vi "Add Lockin Comments.vi"(7 "error in (no error)":errorcluster, 10 "Control Experiment":refnum<class "Control Experiment.lvclass">) -> (0 "error out":errorcluster, 3 "Control Experiment out":refnum<class "Control Experiment.lvclass">)   [LabVIEW 2016, in "Control Experiment.lvclass"]
uses:
  Control Experiment.lvclass
  Typedefs/Lockin Configuration--cluster.ctl
  <userlib>/LevyLab/Lockin-Multichannel/Instrument.Lockin/Typedefs/AO-cluster.ctl
  <userlib>/LevyLab/Lockin-Multichannel/Instrument.Lockin/Typedefs/AO_Amp-array.ctl
  <userlib>/LevyLab/Lockin-Multichannel/Instrument.Lockin/Typedefs/AO_DC-array.ctl
  <userlib>/LevyLab/Lockin-Multichannel/Instrument.Lockin/Typedefs/AO_f-array.ctl
  <userlib>/LevyLab/Lockin-Multichannel/Instrument.Lockin/Typedefs/AO_phi-array.ctl
  <userlib>/LevyLab/Lockin-Multichannel/Instrument.Lockin/Typedefs/Function-array.ctl
  <userlib>/LevyLab/Lockin-Multichannel/Instrument.Lockin/Typedefs/Function-enum.ctl
  <userlib>/LevyLab/Lockin-Multichannel/Instrument.Lockin/Typedefs/REF-cluster.ctl
  <userlib>/LevyLab/Lockin-Multichannel/Instrument.Lockin/Typedefs/REF_f-array.ctl
  <userlib>/LevyLab/Lockin-Multichannel/Instrument.Lockin/Typedefs/REF_phi-array.ctl
  <userlib>/LevyLab/Lockin-Multichannel/Instrument.Lockin/Typedefs/Sampling.ctl
  <userlib>/LevyLab/Lockin-Multichannel/Instrument.Lockin/Typedefs/REF filter-cluster.ctl
  Control Experiment.lvclass/Control Experiment.ctl
  <userlib>/LevyLab/Lockin-Multichannel/Instrument.Lockin/Instrument.Lockin.lvclass
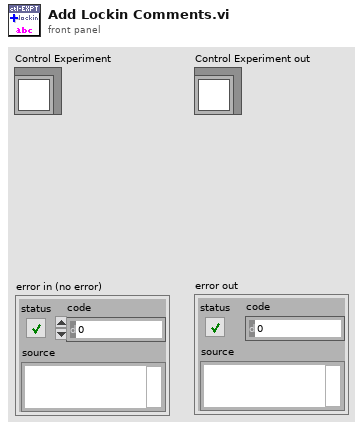
[diagram p1: front panel]
types:
  T1 = typedef "Control Experiment.lvclass/Lockin Configuration--cluster.ctl" = cluster{"Channels: AO":T2, "REF config":T9, "sampling":T12, "REF filter":T13}
  T2 = typedef "Instrument.Lockin.lvclass/AO-cluster.ctl" = cluster{"AO Amp (V)":T3, "AO DC (V)":T4, "AO f (Hz)":T5, "AO Phase (°)":T6, "Function":T7, "I+":bool[], "Sweeping":bool[]}
  T3 = typedef "Instrument.Lockin.lvclass/AO_Amp-array.ctl" = dbl[]
  T4 = typedef "Instrument.Lockin.lvclass/AO_DC-array.ctl" = dbl[]
  T5 = typedef "Instrument.Lockin.lvclass/AO_f-array.ctl" = dbl[]
  T6 = typedef "Instrument.Lockin.lvclass/AO_phi-array.ctl" = dbl[]
  T7 = typedef "Instrument.Lockin.lvclass/Function-array.ctl" = T8[]
  T8 = typedef "Instrument.Lockin.lvclass/Function-enum.ctl" = enum16{"Sine", "Triangle", "Square", "Sawtooth"}
  T9 = typedef "Instrument.Lockin.lvclass/REF-cluster.ctl" = cluster{"REF f (Hz)":T10, "REF phi (°)":T11}
  T10 = typedef "Instrument.Lockin.lvclass/REF_f-array.ctl" = dbl[]
  T11 = typedef "Instrument.Lockin.lvclass/REF_phi-array.ctl" = dbl[]
  T12 = typedef "Instrument.Lockin.lvclass/Sampling.ctl" = cluster{"Fs":i32, "#s":i32}
  T13 = typedef "Instrument.Lockin.lvclass/REF filter-cluster.ctl" = cluster{"TC (s)":dbl, "order":i32}
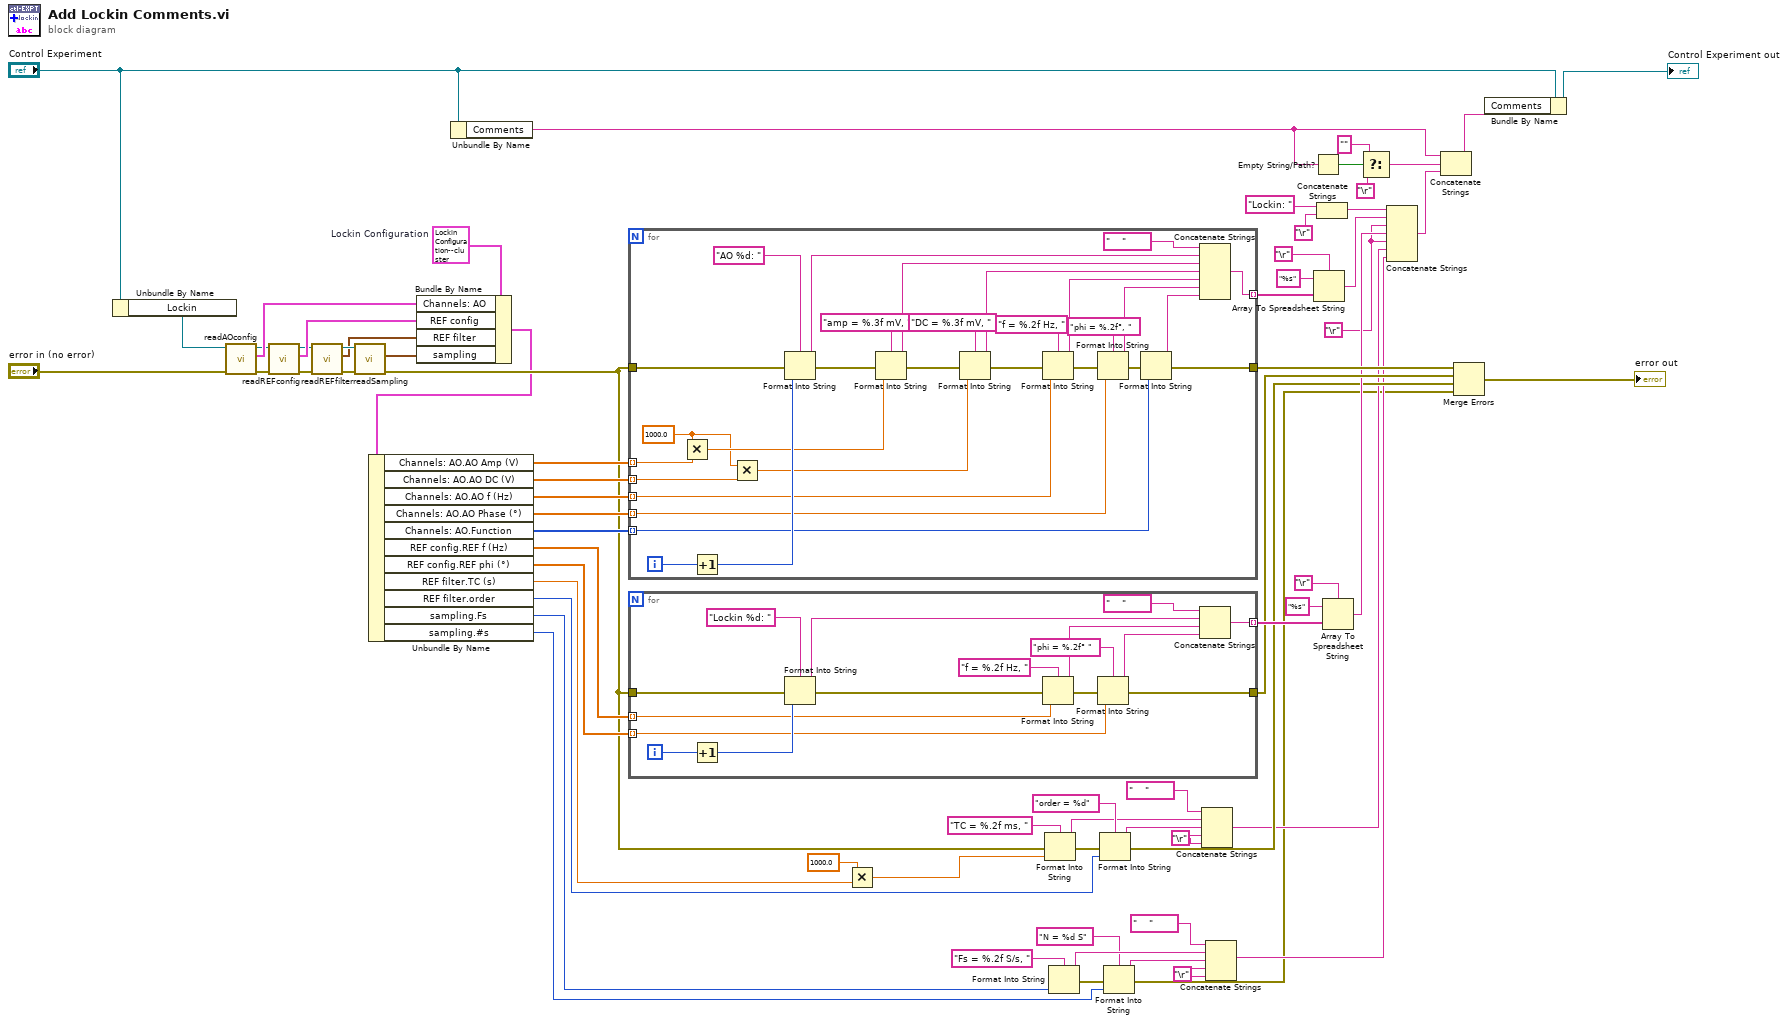
[diagram p0: block diagram]
diagram:
  w17 = T1 {"Channels: AO"={"AO Amp (V)"=[0.01, 0.0, 0.0, 0.0, 0.0, 0.0, 0.0, 0.0], "AO DC (V)"=[0.0, 0.0, 0.0, 0.0, 0.0, 0.0, 0.0, 0.0], "AO f (Hz)"=[13.1, 13.0, 13.0, 13.0, 13.0, 13.0, 13.0, 13.0], "AO Phase (°)"=[0.0, 0.0, 0.0, 0.0, 0.0, 0.0, 0.0, 0.0], "Function"=[enum."Sine", enum."Sine", enum."Sine", enum."Sine", enum."Sine", enum."Sine", enum."Sine", enum."Sine"], "I+"=[], "Sweeping"=[]}, "REF config"={"REF f (Hz)"=[13.0, 26.0], "REF phi (°)"=[0.0, 0.0, 0.0, 0.0, 0.0, 0.0, 0.0, 0.0]}, "sampling"={"Fs"=204789, "#s"=15753}, "REF filter"={"TC (s)"=0.3, "order"=2}}  # Lockin Configuration
  w21 = "\r"
  w24 = "\r"
  w25 = "\r"
  n1 = Unbundle By Name("Control Experiment") -> ("Lockin"=w3:refnum<class "Instrument.Lockin.lvclass">)
  n2 = call <userlib>:"readAOconfig.vi"("error in (no error)"="error in (no error)", "Instrument.Lockin in"=w3) -> ("error out"=w14:errorcluster, "AOconfig"=w11:T2, "Instrument.Lockin out"=w10:refnum<class "Instrument.Lockin.lvclass">)  [unwired: 7 in]
  n3 = call <userlib>:"readREFconfig.vi"("error in (no error)"=w14, "Instrument.Lockin in"=w10) -> ("error out"=w15:errorcluster, "REFconfig"=w12:T9, "Instrument.Lockin out"=w9:refnum<class "Instrument.Lockin.lvclass">)  [unwired: 7 in]
  n4 = call <userlib>:"readREFfilter.vi"("error in (no error)"=w15, "Instrument.Lockin in"=w9) -> ("error out"=w16:errorcluster, "REF filter"=w7:T13, "Instrument.Lockin out"=w8:refnum<class "Instrument.Lockin.lvclass">)  [unwired: 7 in]
  n5 = call <userlib>:"readSampling.vi"("error in (no error)"=w16, "Instrument.Lockin in"=w8) -> ("error out"=w5:errorcluster, "sampling"=w13:T12)  [unwired: 7 in, 1 out]
  n6 = Bundle By Name(cluster=w17, "Channels: AO"=w11, "REF config"=w12, "REF filter"=w7, "sampling"=w13) -> (w2:T1)
  n7 = Unbundle By Name(w2) -> ("Channels: AO.AO Amp (V)"=w66:T3, "Channels: AO.AO DC (V)"=w67:T4, "Channels: AO.AO f (Hz)"=w68:T5, "Channels: AO.AO Phase (°)"=w69:T6, "Channels: AO.Function"=w70:T7, "REF config.REF f (Hz)"=w53:T10, "REF config.REF phi (°)"=w52:T11, "REF filter.TC (s)"=w37:dbl, "REF filter.order"=w39:i32, "sampling.Fs"=w28:i32, "sampling.#s"=w27:i32)
  n8 = Unbundle By Name("Control Experiment") -> ("Comments"=w20:string)
  n9 = for {
    tunnel: w66 -> [w74] mode=indexing
    tunnel: w67 -> [w75] mode=indexing
    tunnel: w68 -> [w83] mode=indexing
    tunnel: w69 -> [w81] mode=indexing
    tunnel: w70 -> [w82] mode=indexing
    tunnel: [w100] -> w63 mode=indexing
    tunnel: w5 -> [w99]
    tunnel: [w94] -> w48
    i -> [w92]
    w71 = 1000.0 ("x")
    n10 = Multiply(x=w71, y=w74) -> (x*y=w72:dbl)
    n11 = Increment(x=w92) -> (x+1=w86:i32)
    n12 = Multiply(x=w71, y=w75) -> (x*y=w73:dbl)
    n13 = Format Into String(format string="AO %d: ", error in=w99, w86) -> (resulting string=w89:string, error out=w98:errorcluster)  [unwired: 1 in]
    n14 = Format Into String(format string="amp = %.3f mV, ", error in=w98, w72) -> (resulting string=w88:string, error out=w93:errorcluster)  [unwired: 1 in]
    n15 = Format Into String(format string="DC = %.3f mV, ", error in=w93, w73) -> (resulting string=w85:string, error out=w97:errorcluster)  [unwired: 1 in]
    n16 = Format Into String(format string="f = %.2f Hz, ", error in=w97, w83) -> (resulting string=w80:string, error out=w96:errorcluster)  [unwired: 1 in]
    n17 = Format Into String(format string="phi = %.2f°, ", error in=w96, w81) -> (resulting string=w78:string, error out=w95:errorcluster)  [unwired: 1 in]
    n18 = Format Into String(error in=w95, w82) -> (resulting string=w77:string, error out=w94:errorcluster)  [unwired: 2 in]
    n19 = Concatenate Strings("    " ("string"), w89, w88, w85, w80, w78, w77) -> (w100:string)
  }
  n20 = for {
    tunnel: w53 -> [w108] mode=indexing
    tunnel: w52 -> [w107] mode=indexing
    tunnel: [w116] -> w49 mode=indexing
    tunnel: w5 -> [w115]
    tunnel: [w102] -> w47
    i -> [w113]
    n21 = Increment(x=w113) -> (x+1=w110:i32)
    n22 = Format Into String(format string="Lockin %d: ", error in=w115, w110) -> (resulting string=w111:string, error out=w103:errorcluster)  [unwired: 1 in]
    n23 = Format Into String(format string="f = %.2f Hz, ", error in=w103, w108) -> (resulting string=w106:string, error out=w114:errorcluster)  [unwired: 1 in]
    n24 = Format Into String(format string="phi = %.2f° ", error in=w114, w107) -> (resulting string=w105:string, error out=w102:errorcluster)  [unwired: 1 in]
    n25 = Concatenate Strings("    " ("string"), w111, w106, w105) -> (w116:string)
  }
  n26 = Multiply(x=1000.0, y=w37) -> (x*y=w36:dbl)
  n27 = Format Into String(format string="TC = %.2f ms, ", error in=w5, w36) -> (resulting string=w42:string, error out=w40:errorcluster)  [unwired: 1 in]
  n28 = Format Into String(format string="Fs = %.2f S/s, ", w28) -> (resulting string=w31:string, error out=w33:errorcluster)  [unwired: 2 in]
  n29 = Format Into String(format string="order = %d", error in=w40, w39) -> (resulting string=w43:string, error out=w35:errorcluster)  [unwired: 1 in]
  n30 = Format Into String(format string="N = %d S", error in=w33, w27) -> (resulting string=w30:string, error out=w1:errorcluster)  [unwired: 1 in]
  n31 = Concatenate Strings("    " ("string"), w42, w43, w25, w25) -> (w22:string)
  n32 = Concatenate Strings("    " ("string"), w31, w30, w24, w24) -> (w23:string)
  n33 = Empty String/Path?(string/path=w20) -> (empty?=w57:bool)
  n34 = Array To Spreadsheet String(delimiter (Tab)="\r", array=w63, 3:"%s" ("format string")) -> (spreadsheet string=w59:string)
  n35 = Concatenate Strings("Lockin: " ("string"), "\r") -> (w60:string)
  n36 = Array To Spreadsheet String(delimiter (Tab)="\r", array=w49, 3:"%s" ("format string")) -> (spreadsheet string=w45:string)
  n37 = Select(t="", s=w57, f="\r") -> (s? t:f=w54:string)
  n38 = Concatenate Strings(w60, w59, w21, w45, w21, w22, w23) -> (w58:string)
  n39 = Concatenate Strings(w20, w54, w58) -> (w18:string)
  n40 = Merge Errors(w48, w47, w35, w1) -> (→"error out":errorcluster)
  n41 = Bundle By Name(cluster="Control Experiment", "Comments"=w18) -> (→"Control Experiment out":refnum<class "Control Experiment.lvclass">)
